vi "Read Test Configuration (INI) File_MultiTest.vi"() -> (1 "Filename":string, 2 "Filepath":path, 3 "Experiments":T2={"Exp 1"={"Floor_Sweep_Stop_V"=36.0, "Resistance Threshold"=1.0, "Floor_Sweep_Start_V"=36.0, "Floor_Sweep_Step_V"=1.0, "Roof_Sweep_Stop_V"=36.0, "Roof_Sweep_Start_V"=36.0, "Roof_Sweep_Step_V"=1.0, "Experiment Name"="", "Meas_Type"=[0, 2, 4]}, "Exp 2"={"Floor_Sweep_Stop_V"=36.0, "Resistance Threshold"=1.0, "Floor_Sweep_Start_V"=36.0, "Floor_Sweep_Step_V"=1.0, "Roof_Sweep_Stop_V"=36.0, "Roof_Sweep_Start_V"=36.0, "Roof_Sweep_Step_V"=1.0, "Experiment Name"="", "Meas_Type"=[0, 2, 4]}, "Exp 3"={"Floor_Sweep_Stop_V"=36.0, "Resistance Threshold"=1.0, "Floor_Sweep_Start_V"=36.0, "Floor_Sweep_Step_V"=1.0, "Roof_Sweep_Stop_V"=36.0, "Roof_Sweep_Start_V"=36.0, "Roof_Sweep_Step_V"=1.0, "Experiment Name"="", "Meas_Type"=[0, 2, 4]}, "Exp 4"={"Floor_Sweep_Stop_V"=36.0, "Resistance Threshold"=1.0, "Floor_Sweep_Start_V"=36.0, "Floor_Sweep_Step_V"=1.0, "Roof_Sweep_Stop_V"=36.0, "Roof_Sweep_Start_V"=36.0, "Roof_Sweep_Step_V"=1.0, "Experiment Name"="", "Meas_Type"=[0, 2, 4]}}, 4 "ListBox_Selected_Tests":T1, 5 "# of Cycles":string)   [LabVIEW 2013]
doc: "Read Test Configuration file. Set Cluster Output which SDR will choose from later."
uses:
  Support/Controls/Multiple Exp Setup_MultiTest.ctl
  Support/Controls/Individual User Inputs_MultiTest.ctl
  Support/Controls/Test Selection.ctl
  <vilib>/Utility/config.llb/Read Key (String).vi
  <vilib>/Utility/config.llb/Read Key (Double).vi
  <vilib>/Utility/config.llb/Read Key (Path).vi
  <vilib>/Utility/config.llb/NI_LVConfig.lvlib
panel:
  # "Calculation Settings"
  # "Test Settings"
  # "Calculation Settings"
  # "Test Settings"
  # "Calculation Settings"
  # "Test Settings"
  # "Calculation Settings"
  # "Test Settings"
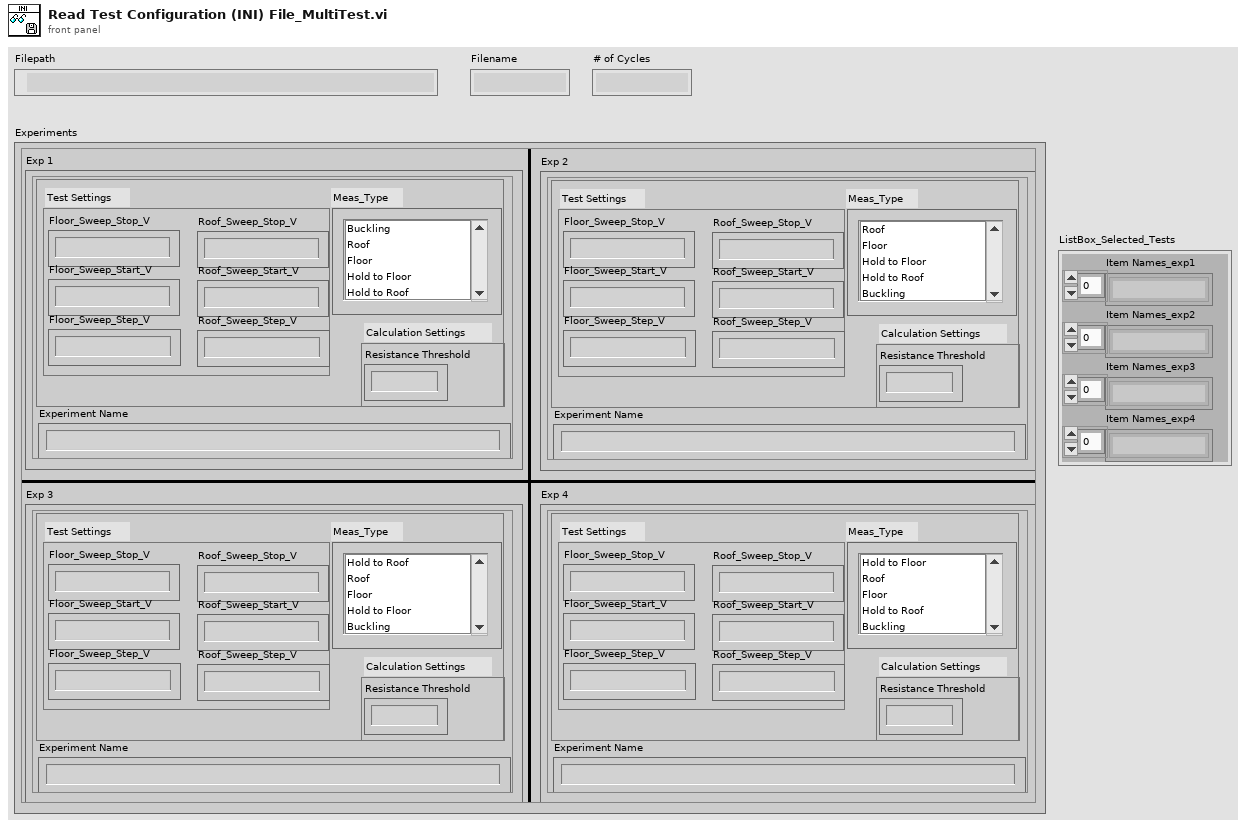
[diagram p1: front panel]
types:
  T1 = cluster{"Item Names_exp1":string[], "Item Names_exp2":string[], "Item Names_exp3":string[], "Item Names_exp4":string[]}
  T2 = typedef "Multiple Exp Setup_MultiTest.ctl" = cluster{"Exp 1":T3, "Exp 2":T3, "Exp 3":T3, "Exp 4":T3}
  T3 = typedef "Individual User Inputs_MultiTest.ctl" = cluster{"Floor_Sweep_Stop_V":dbl, "Resistance Threshold":dbl, "Floor_Sweep_Start_V":dbl, "Floor_Sweep_Step_V":dbl, "Roof_Sweep_Stop_V":dbl, "Roof_Sweep_Start_V":dbl, "Roof_Sweep_Step_V":dbl, "Experiment Name":string, "Meas_Type":T4}
  T4 = typedef "Test Selection.ctl" = i32[]
  T5 = typedef "NI_LVConfig.lvlib/Config Data RefNum.ctl" = refnum<k1>
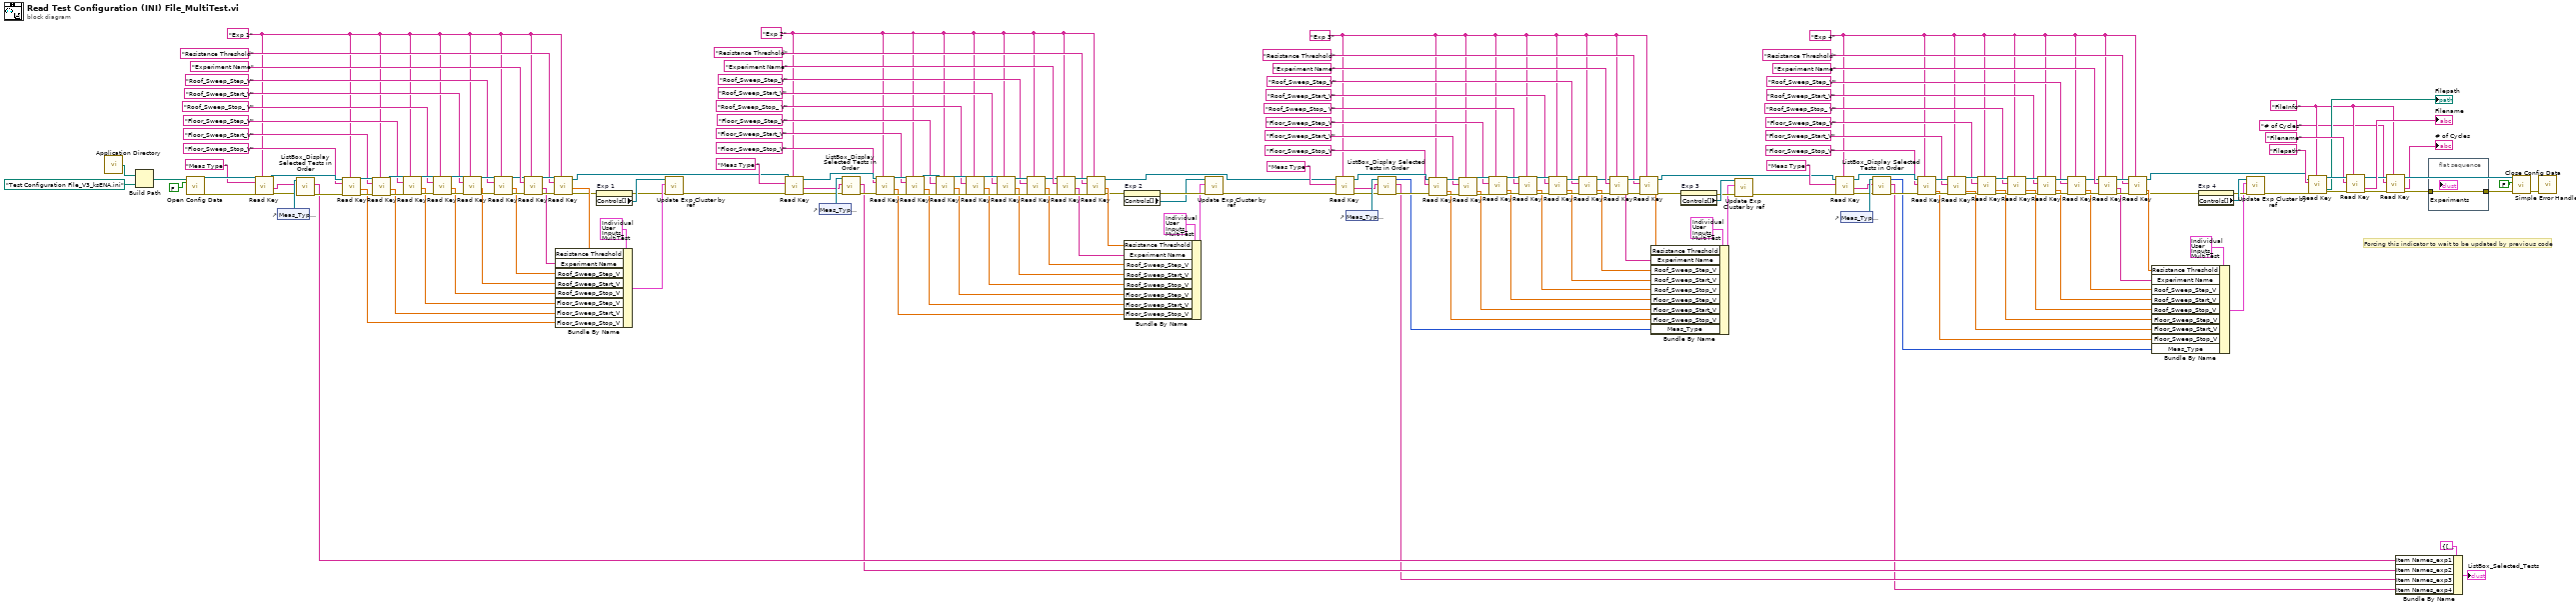
[diagram p0: block diagram]
diagram:
  w62 = "FileInfo" ("section")
  w83 = "Exp 4" ("section")
  w117 = "Exp 3" ("section")
  w151 = "Exp 2" ("section")
  w176 = "Exp 1" ("section")
  # "Forcing this indicator to wait to be updated by previous code"
  n1 = call <vilib>:"Application Directory.vi"() -> ("Application Directory"=w197:path)
  n2 = Build Path(base path=w197, name or relative path=path "Test Configuration File_V3_ksENA.ini" ("default name")) -> (appended path=w204:path)
  n3 = call <vilib>:"Open Config Data.vi"("create file if necessary (T)"=FALSE ("create file if necessary? (T)"), "configuration file path"=w204) -> ("error out"=w192:errorcluster, "refnum"=w193:T5)  [unwired: 7 in, 1 out]
  n4 = call-poly <vilib>:"Read Key.vi"("section"=w176, "error in (no error)"=w192, "key"="Meas Type " ("Key 1"), "refnum"=w193) -> ("error out"=w55:errorcluster, "value"=w44:string, "refnum out"=w194:T5)  [unwired: 4 in, 1 out]
  n5 = control-ref of="Meas_Type_exp1"() -> (w59:refnum<vi>)
  n6 = call "ListBox_Display Selected Tests in Order.vi"("Error In"=w55, "Tests"=w44, "Meas_Type_exp1"=w59) -> ("Error Out"=w54:errorcluster, "Item Names"=w38:string[])  [unwired: 6 in, 1 out]
  n7 = call-poly <vilib>:"Read Key.vi"("section"=w176, "error in (no error)"=w54, "key"="Floor_Sweep_Stop_V" ("Key 2"), "refnum"=w194) -> ("error out"=w196:errorcluster, "value"=w33:dbl, "refnum out"=w195:T5)  [unwired: 4 in, 1 out]
  n8 = call-poly <vilib>:"Read Key.vi"("section"=w176, "error in (no error)"=w196, "key"="Floor_Sweep_Start_V" ("Key 2"), "refnum"=w195) -> ("error out"=w201:errorcluster, "value"=w32:dbl, "refnum out"=w200:T5)  [unwired: 4 in, 1 out]
  n9 = call-poly <vilib>:"Read Key.vi"("section"=w176, "error in (no error)"=w201, "key"="Floor_Sweep_Step_V" ("Key 2"), "refnum"=w200) -> ("error out"=w202:errorcluster, "value"=w31:dbl, "refnum out"=w203:T5)  [unwired: 1 in, 4 out]
  n10 = call-poly <vilib>:"Read Key.vi"("section"=w176, "error in (no error)"=w202, "key"="Roof_Sweep_Stop_ V" ("Key 3"), "refnum"=w203) -> ("error out"=w199:errorcluster, "value"=w30:dbl, "refnum out"=w198:T5)  [unwired: 1 in, 4 out]
  n11 = call-poly <vilib>:"Read Key.vi"("section"=w176, "error in (no error)"=w199, "key"="Roof_Sweep_Start_V" ("Key 3"), "refnum"=w198) -> ("error out"=w182:errorcluster, "value"=w29:dbl, "refnum out"=w183:T5)  [unwired: 1 in, 4 out]
  n12 = call-poly <vilib>:"Read Key.vi"("section"=w176, "error in (no error)"=w182, "key"="Roof_Sweep_Step_V" ("Key 3"), "refnum"=w183) -> ("error out"=w185:errorcluster, "value"=w28:dbl, "refnum out"=w178:T5)  [unwired: 1 in, 4 out]
  n13 = call-poly <vilib>:"Read Key.vi"("section"=w176, "error in (no error)"=w185, "key"="Experiment Name" ("Key 3"), "refnum"=w178) -> ("error out"=w184:errorcluster, "value"=w27:string, "refnum out"=w179:T5)  [unwired: 2 in, 3 out]
  n14 = call-poly <vilib>:"Read Key.vi"("section"=w176, "error in (no error)"=w184, "key"="Resistance Threshold" ("Key 3"), "refnum"=w179) -> ("error out"=w17:errorcluster, "value"=w26:dbl, "refnum out"=w150:T5)  [unwired: 2 in, 3 out]
  n15 = Bundle By Name(cluster=T3 {"Floor_Sweep_Stop_V"=5.0, "Resistance Threshold"=1000.0, "Floor_Sweep_Start_V"=0.0, "Floor_Sweep_Step_V"=1.0, "Roof_Sweep_Stop_V"=5.0, "Roof_Sweep_Start_V"=0.0, "Roof_Sweep_Step_V"=1.0, "Experiment Name"="", "Meas_Type"=[0]} ("Exp 1"), "Resistance Threshold"=w26, "Experiment Name"=w27, "Roof_Sweep_Step_V"=w28, "Roof_Sweep_Start_V"=w29, "Roof_Sweep_Stop_V"=w30, "Floor_Sweep_Step_V"=w31, "Floor_Sweep_Start_V"=w32, "Floor_Sweep_Stop_V"=w33) -> (w24:T3)
  n16 = property on="Exp 1" class="Clust (strict)"(error in=w17) -> (error out=w16:errorcluster, "Controls[]"=w34:refnum<vi>[])  [unwired: 1 in, 1 out]
  n17 = call "Update Exp Cluster by ref.vi"("Error In"=w16, "Exp 1"=w24, "Controls[]"=w34) -> ("Error Out"=w18:errorcluster)  [unwired: 8 in]
  n18 = call-poly <vilib>:"Read Key.vi"("section"=w151, "error in (no error)"=w18, "key"="Meas Type " ("Key 1"), "refnum"=w150) -> ("error out"=w53:errorcluster, "value"=w43:string, "refnum out"=w167:T5)  [unwired: 4 in, 1 out]
  n19 = control-ref of="Meas_Type_exp2"() -> (w58:refnum<vi>)
  n20 = call "ListBox_Display Selected Tests in Order.vi"("Error In"=w53, "Tests"=w43, "Meas_Type_exp1"=w58) -> ("Error Out"=w52:errorcluster, "Item Names"=w37:string[])  [unwired: 6 in, 1 out]
  n21 = call-poly <vilib>:"Read Key.vi"("section"=w151, "error in (no error)"=w52, "key"="Floor_Sweep_Stop_V" ("Key 2"), "refnum"=w167) -> ("error out"=w169:errorcluster, "value"=w142:dbl, "refnum out"=w168:T5)  [unwired: 4 in, 1 out]
  n22 = call-poly <vilib>:"Read Key.vi"("section"=w151, "error in (no error)"=w169, "key"="Floor_Sweep_Start_V" ("Key 2"), "refnum"=w168) -> ("error out"=w173:errorcluster, "value"=w143:dbl, "refnum out"=w172:T5)  [unwired: 4 in, 1 out]
  n23 = call-poly <vilib>:"Read Key.vi"("section"=w151, "error in (no error)"=w173, "key"="Floor_Sweep_Step_V" ("Key 2"), "refnum"=w172) -> ("error out"=w174:errorcluster, "value"=w144:dbl, "refnum out"=w175:T5)  [unwired: 1 in, 4 out]
  n24 = call-poly <vilib>:"Read Key.vi"("section"=w151, "error in (no error)"=w174, "key"="Roof_Sweep_Stop_ V" ("Key 3"), "refnum"=w175) -> ("error out"=w171:errorcluster, "value"=w145:dbl, "refnum out"=w170:T5)  [unwired: 1 in, 4 out]
  n25 = call-poly <vilib>:"Read Key.vi"("section"=w151, "error in (no error)"=w171, "key"="Roof_Sweep_Start_V" ("Key 3"), "refnum"=w170) -> ("error out"=w157:errorcluster, "value"=w146:dbl, "refnum out"=w158:T5)  [unwired: 1 in, 4 out]
  n26 = call-poly <vilib>:"Read Key.vi"("section"=w151, "error in (no error)"=w157, "key"="Roof_Sweep_Step_V" ("Key 3"), "refnum"=w158) -> ("error out"=w160:errorcluster, "value"=w147:dbl, "refnum out"=w153:T5)  [unwired: 1 in, 4 out]
  n27 = call-poly <vilib>:"Read Key.vi"("section"=w151, "error in (no error)"=w160, "key"="Experiment Name" ("Key 3"), "refnum"=w153) -> ("error out"=w159:errorcluster, "value"=w148:string, "refnum out"=w154:T5)  [unwired: 2 in, 3 out]
  n28 = call-poly <vilib>:"Read Key.vi"("section"=w151, "error in (no error)"=w159, "key"="Resistance Threshold" ("Key 3"), "refnum"=w154) -> ("error out"=w14:errorcluster, "value"=w149:dbl, "refnum out"=w116:T5)  [unwired: 2 in, 3 out]
  n29 = Bundle By Name(cluster=T3 {"Floor_Sweep_Stop_V"=5.0, "Resistance Threshold"=1000.0, "Floor_Sweep_Start_V"=0.0, "Floor_Sweep_Step_V"=1.0, "Roof_Sweep_Stop_V"=5.0, "Roof_Sweep_Start_V"=0.0, "Roof_Sweep_Step_V"=1.0, "Experiment Name"="", "Meas_Type"=[0]} ("Exp 1"), "Resistance Threshold"=w149, "Experiment Name"=w148, "Roof_Sweep_Step_V"=w147, "Roof_Sweep_Start_V"=w146, "Roof_Sweep_Stop_V"=w145, "Floor_Sweep_Step_V"=w144, "Floor_Sweep_Start_V"=w143, "Floor_Sweep_Stop_V"=w142) -> (w11:T3)
  n30 = property on="Exp 2" class="Clust (strict)"(error in=w14) -> (error out=w15:errorcluster, "Controls[]"=w12:refnum<vi>[])  [unwired: 1 in, 1 out]
  n31 = call "Update Exp Cluster by ref.vi"("Error In"=w15, "Exp 1"=w11, "Controls[]"=w12) -> ("Error Out"=w13:errorcluster)  [unwired: 8 in]
  n32 = call-poly <vilib>:"Read Key.vi"("section"=w117, "error in (no error)"=w13, "key"="Meas Type " ("Key 1"), "refnum"=w116) -> ("error out"=w51:errorcluster, "value"=w42:string, "refnum out"=w133:T5)  [unwired: 4 in, 1 out]
  n33 = control-ref of="Meas_Type_exp3"() -> (w57:refnum<vi>)
  n34 = call "ListBox_Display Selected Tests in Order.vi"("Error In"=w51, "Tests"=w42, "Meas_Type_exp1"=w57) -> ("Error Out"=w50:errorcluster, "Item Names"=w36:string[], "Values"=w47:i32[])  [unwired: 6 in]
  n35 = call-poly <vilib>:"Read Key.vi"("section"=w117, "error in (no error)"=w50, "key"="Floor_Sweep_Stop_V" ("Key 2"), "refnum"=w133) -> ("error out"=w135:errorcluster, "value"=w108:dbl, "refnum out"=w134:T5)  [unwired: 4 in, 1 out]
  n36 = call-poly <vilib>:"Read Key.vi"("section"=w117, "error in (no error)"=w135, "key"="Floor_Sweep_Start_V" ("Key 2"), "refnum"=w134) -> ("error out"=w139:errorcluster, "value"=w109:dbl, "refnum out"=w138:T5)  [unwired: 4 in, 1 out]
  n37 = call-poly <vilib>:"Read Key.vi"("section"=w117, "error in (no error)"=w139, "key"="Floor_Sweep_Step_V" ("Key 2"), "refnum"=w138) -> ("error out"=w140:errorcluster, "value"=w110:dbl, "refnum out"=w141:T5)  [unwired: 1 in, 4 out]
  n38 = call-poly <vilib>:"Read Key.vi"("section"=w117, "error in (no error)"=w140, "key"="Roof_Sweep_Stop_ V" ("Key 3"), "refnum"=w141) -> ("error out"=w137:errorcluster, "value"=w111:dbl, "refnum out"=w136:T5)  [unwired: 1 in, 4 out]
  n39 = call-poly <vilib>:"Read Key.vi"("section"=w117, "error in (no error)"=w137, "key"="Roof_Sweep_Start_V" ("Key 3"), "refnum"=w136) -> ("error out"=w123:errorcluster, "value"=w112:dbl, "refnum out"=w124:T5)  [unwired: 1 in, 4 out]
  n40 = call-poly <vilib>:"Read Key.vi"("section"=w117, "error in (no error)"=w123, "key"="Roof_Sweep_Step_V" ("Key 3"), "refnum"=w124) -> ("error out"=w126:errorcluster, "value"=w113:dbl, "refnum out"=w119:T5)  [unwired: 1 in, 4 out]
  n41 = call-poly <vilib>:"Read Key.vi"("section"=w117, "error in (no error)"=w126, "key"="Experiment Name" ("Key 3"), "refnum"=w119) -> ("error out"=w125:errorcluster, "value"=w114:string, "refnum out"=w120:T5)  [unwired: 2 in, 3 out]
  n42 = call-poly <vilib>:"Read Key.vi"("section"=w117, "error in (no error)"=w125, "key"="Resistance Threshold" ("Key 3"), "refnum"=w120) -> ("error out"=w8:errorcluster, "value"=w115:dbl, "refnum out"=w82:T5)  [unwired: 2 in, 3 out]
  n43 = Bundle By Name(cluster=T3 {"Floor_Sweep_Stop_V"=5.0, "Resistance Threshold"=1000.0, "Floor_Sweep_Start_V"=0.0, "Floor_Sweep_Step_V"=1.0, "Roof_Sweep_Stop_V"=5.0, "Roof_Sweep_Start_V"=0.0, "Roof_Sweep_Step_V"=1.0, "Experiment Name"="", "Meas_Type"=[0]} ("Exp 1"), "Resistance Threshold"=w115, "Experiment Name"=w114, "Roof_Sweep_Step_V"=w113, "Roof_Sweep_Start_V"=w112, "Roof_Sweep_Stop_V"=w111, "Floor_Sweep_Step_V"=w110, "Floor_Sweep_Start_V"=w109, "Floor_Sweep_Stop_V"=w108, "Meas_Type"=w47) -> (w6:T3)
  n44 = property on="Exp 3" class="Clust (strict)"(error in=w8) -> (error out=w9:errorcluster, "Controls[]"=w10:refnum<vi>[])  [unwired: 1 in, 1 out]
  n45 = call "Update Exp Cluster by ref.vi"("Error In"=w9, "Exp 1"=w6, "Controls[]"=w10) -> ("Error Out"=w7:errorcluster)  [unwired: 8 in]
  n46 = call-poly <vilib>:"Read Key.vi"("section"=w83, "error in (no error)"=w7, "key"="Meas Type " ("Key 1"), "refnum"=w82) -> ("error out"=w49:errorcluster, "value"=w41:string, "refnum out"=w99:T5)  [unwired: 4 in, 1 out]
  n47 = control-ref of="Meas_Type_exp4"() -> (w56:refnum<vi>)
  n48 = call "ListBox_Display Selected Tests in Order.vi"("Error In"=w49, "Tests"=w41, "Meas_Type_exp1"=w56) -> ("Error Out"=w48:errorcluster, "Item Names"=w35:string[], "Values"=w46:i32[])  [unwired: 6 in]
  n49 = call-poly <vilib>:"Read Key.vi"("section"=w83, "error in (no error)"=w48, "key"="Floor_Sweep_Stop_V" ("Key 2"), "refnum"=w99) -> ("error out"=w101:errorcluster, "value"=w74:dbl, "refnum out"=w100:T5)  [unwired: 4 in, 1 out]
  n50 = call-poly <vilib>:"Read Key.vi"("section"=w83, "error in (no error)"=w101, "key"="Floor_Sweep_Start_V" ("Key 2"), "refnum"=w100) -> ("error out"=w105:errorcluster, "value"=w75:dbl, "refnum out"=w104:T5)  [unwired: 4 in, 1 out]
  n51 = call-poly <vilib>:"Read Key.vi"("section"=w83, "error in (no error)"=w105, "key"="Floor_Sweep_Step_V" ("Key 2"), "refnum"=w104) -> ("error out"=w106:errorcluster, "value"=w76:dbl, "refnum out"=w107:T5)  [unwired: 1 in, 4 out]
  n52 = call-poly <vilib>:"Read Key.vi"("section"=w83, "error in (no error)"=w106, "key"="Roof_Sweep_Stop_ V" ("Key 3"), "refnum"=w107) -> ("error out"=w103:errorcluster, "value"=w77:dbl, "refnum out"=w102:T5)  [unwired: 1 in, 4 out]
  n53 = call-poly <vilib>:"Read Key.vi"("section"=w83, "error in (no error)"=w103, "key"="Roof_Sweep_Start_V" ("Key 3"), "refnum"=w102) -> ("error out"=w89:errorcluster, "value"=w78:dbl, "refnum out"=w90:T5)  [unwired: 1 in, 4 out]
  n54 = call-poly <vilib>:"Read Key.vi"("section"=w83, "error in (no error)"=w89, "key"="Roof_Sweep_Step_V" ("Key 3"), "refnum"=w90) -> ("error out"=w92:errorcluster, "value"=w79:dbl, "refnum out"=w85:T5)  [unwired: 1 in, 4 out]
  n55 = call-poly <vilib>:"Read Key.vi"("section"=w83, "error in (no error)"=w92, "key"="Experiment Name" ("Key 3"), "refnum"=w85) -> ("error out"=w91:errorcluster, "value"=w80:string, "refnum out"=w86:T5)  [unwired: 2 in, 3 out]
  n56 = call-poly <vilib>:"Read Key.vi"("section"=w83, "error in (no error)"=w91, "key"="Resistance Threshold" ("Key 3"), "refnum"=w86) -> ("error out"=w5:errorcluster, "value"=w81:dbl, "refnum out"=w66:T5)  [unwired: 2 in, 3 out]
  n57 = Bundle By Name(cluster=T3 {"Floor_Sweep_Stop_V"=5.0, "Resistance Threshold"=1000.0, "Floor_Sweep_Start_V"=0.0, "Floor_Sweep_Step_V"=1.0, "Roof_Sweep_Stop_V"=5.0, "Roof_Sweep_Start_V"=0.0, "Roof_Sweep_Step_V"=1.0, "Experiment Name"="", "Meas_Type"=[0]} ("Exp 1"), "Resistance Threshold"=w81, "Experiment Name"=w80, "Roof_Sweep_Step_V"=w79, "Roof_Sweep_Start_V"=w78, "Roof_Sweep_Stop_V"=w77, "Floor_Sweep_Step_V"=w76, "Floor_Sweep_Start_V"=w75, "Floor_Sweep_Stop_V"=w74, "Meas_Type"=w46) -> (w1:T3)
  n58 = property on="Exp 4" class="Clust (strict)"(error in=w5) -> (error out=w3:errorcluster, "Controls[]"=w4:refnum<vi>[])  [unwired: 1 in, 1 out]
  n59 = call "Update Exp Cluster by ref.vi"("Error In"=w3, "Exp 1"=w1, "Controls[]"=w4) -> ("Error Out"=w2:errorcluster)  [unwired: 8 in]
  n60 = call-poly <vilib>:"Read Key.vi"("section"=w62, "error in (no error)"=w2, "key"="Filepath" ("Key 1"), "refnum"=w66) -> ("error out"=w70:errorcluster, "value"=→"Filepath":path, "refnum out"=w71:T5)  [unwired: 4 in, 1 out]
  n61 = call-poly <vilib>:"Read Key.vi"("section"=w62, "error in (no error)"=w70, "key"="Filename" ("Key 1"), "refnum"=w71) -> ("error out"=w63:errorcluster, "value"=→"Filename":string, "refnum out"=w65:T5)  [unwired: 4 in, 1 out]
  n62 = call-poly <vilib>:"Read Key.vi"("section"=w62, "error in (no error)"=w63, "key"="# of Cycles" ("Key 1"), "refnum"=w65) -> ("error out"=w20:errorcluster, "value"=→"# of Cycles":string, "refnum out"=w64:T5)  [unwired: 4 in, 1 out]
  n63 = Bundle By Name(cluster=T1 {"Item Names_exp1"=[], "Item Names_exp2"=[], "Item Names_exp3"=[], "Item Names_exp4"=[]} ("ListBox_Selected_Tests"), "Item Names_exp1"=w38, "Item Names_exp2"=w37, "Item Names_exp3"=w36, "Item Names_exp4"=w35) -> (→"ListBox_Selected_Tests":T1)
  n64 = flat-sequence {
    tunnel: w20 -> [w207]
    tunnel: [w207] -> w19
    frame #0 {
    }
  }
  n65 = call <vilib>:"Close Config Data.vi"("error in (no error)"=w19, "write file if changed (T)"=FALSE ("write configuration file? (T)"), "refnum"=w64) -> ("error out"=w45:errorcluster)  [unwired: 8 out]
  n66 = call <vilib>:"Simple Error Handler.vi"("error in (no error)"=w45) -> ()  [unwired: 4 in, 5 out]
